vi "type_maintenace.vi"(4 "durée":string, 5 "technicien":string, 6 "Remarque":string, 7 "type":string, 8 "Error in (no error)":errorcluster, 9 "taches_principales":string, 10 "type_description":string, 11 "Connection In":refnum<k7>) -> (0 "Error out":errorcluster, 3 "Connection Out":refnum<k7>)   [LabVIEW 2019]
panel:
  out "concatenated string":string
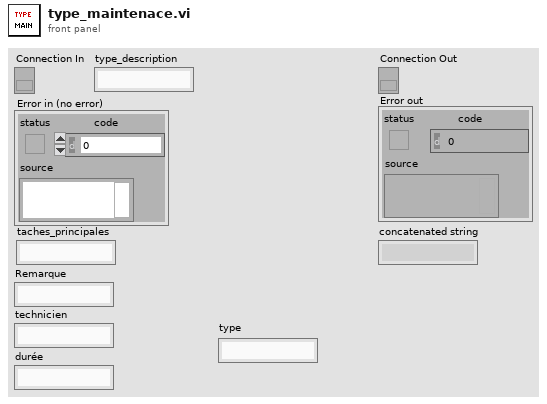
[diagram p1: front panel]
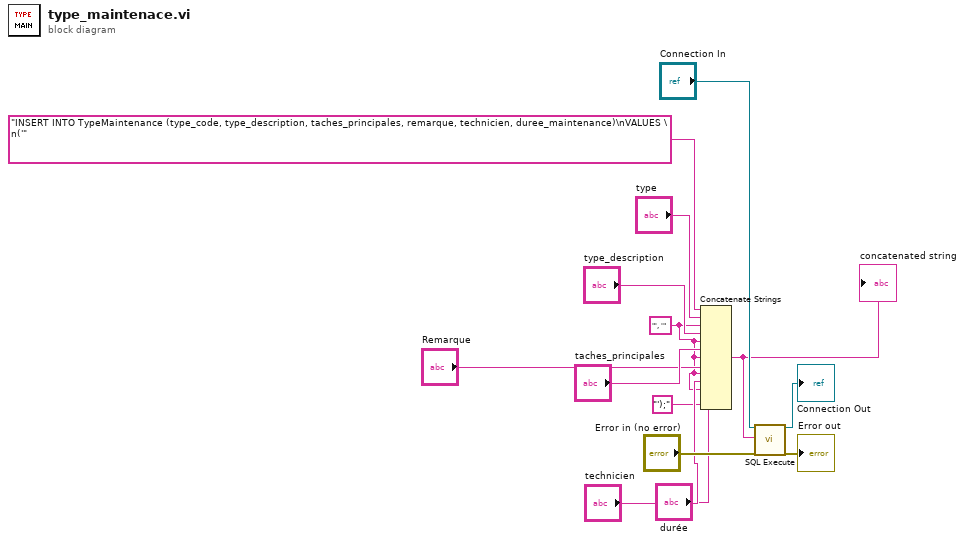
[diagram p0: block diagram]
diagram:
  w3 = "', '" ("string")
  n1 = Concatenate Strings("INSERT INTO TypeMaintenance (type_code, type_description, taches_principales, remarque, technicien, duree_maintenance)\nVALUES \n('" ("SQL Query"), "type", w3, "type_description", w3, "taches_principales", w3, "Remarque", w3, "technicien", w3, "durée", "');" ("string")) -> (w9:string)
  "concatenated string" <- w9
  n2 = call <vilib>:"SQL Execute.vi"("Connection In"="Connection In", "SQL Query"=w9, "Error in (no error)"="Error in (no error)") -> ("Connection Out"=→"Connection Out":refnum<k7>, "Error out"=→"Error out":errorcluster)  [unwired: 15 in]
